vi "Detector - subvi.vi"(8 "error in (no error)":errorcluster) -> (0 "error out":errorcluster, 1 "Total Pixels":i32, 2 "Y Pixels":i32, 3 "X Pixels":i32)   [LabVIEW 2014]
uses:
  Library Files - Andor and MadCity/Andorlib/atmcd32d.lvlib
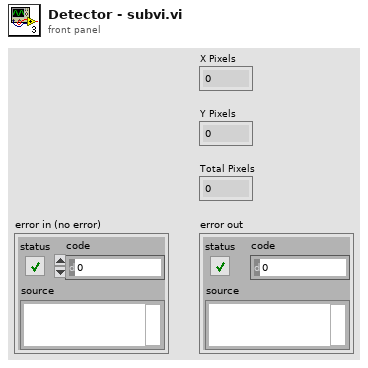
[diagram p1: front panel]
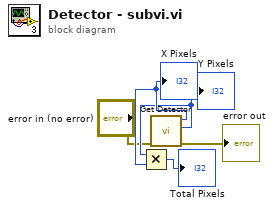
[diagram p0: block diagram]
diagram:
  n1 = call "Get Detector.vi"("error in (no error)"="error in (no error)") -> ("error out"=→"error out":errorcluster, "ypixels out"=w4:i32, "xpixels out"=w5:i32)  [unwired: 7 in, 1 out]
  "Y Pixels" <- w4
  "X Pixels" <- w5
  n2 = Multiply(x=w4, y=w5) -> (x*y=→"Total Pixels":i32)
